vi "FeedTest.vi"(11 "Feed":T1(plugin-control)) -> ()   [LabVIEW 2016]
panel:
  out "Image":T1(plugin-control)
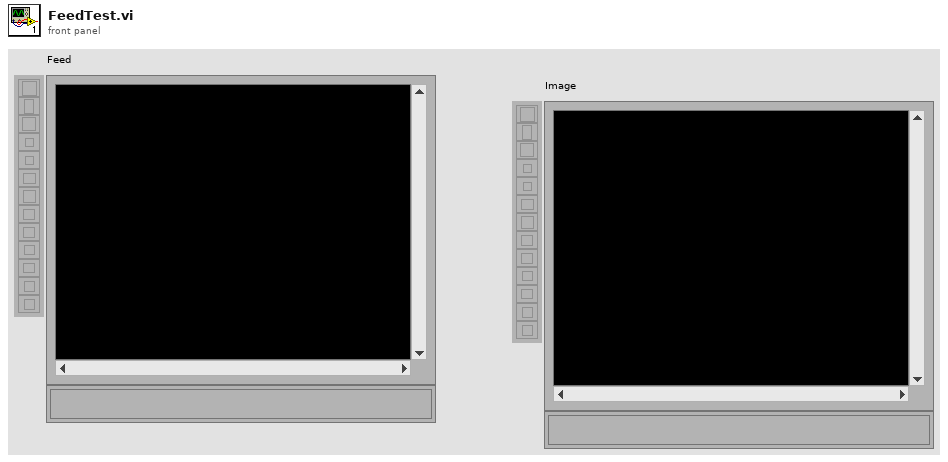
[diagram p1: front panel]
types:
  T1 = typedef "IMAQ Image.ctl" = refnum<image>
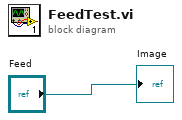
[diagram p0: block diagram]
diagram:
  "Image" <- "Feed"
